vi "GetDefaultAcquisitionFileNames-subvi.vi"(0 "RAID root path":path=path "c:/scratch", 2 "Error In":errorcluster) -> (3 "last directory path":path, 4 "next directory path":path, 5 "all directory names":string[](array[string]), 6 "Error Out":errorcluster)   [LabVIEW 2014]
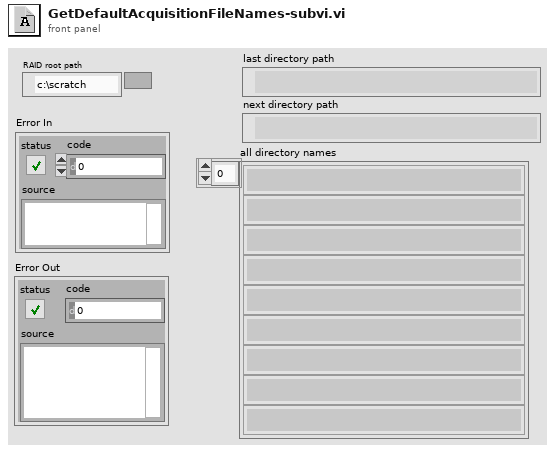
[diagram p1: front panel]
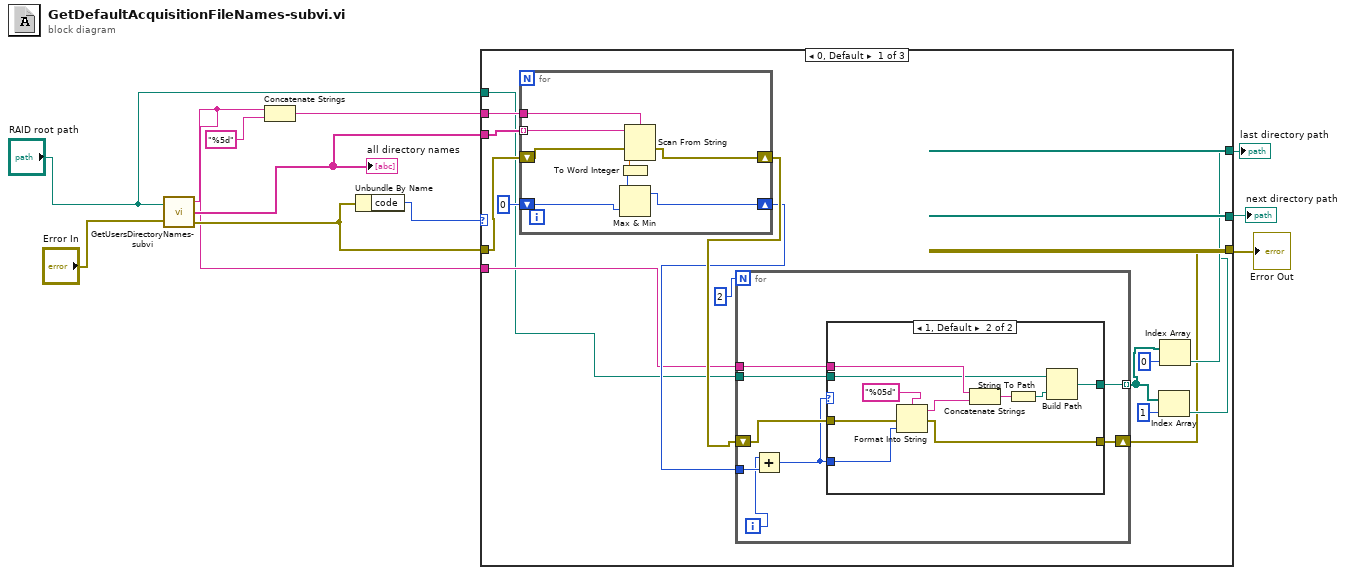
[diagram p0: block diagram]
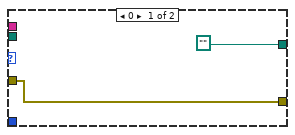
[diagram p2: hidden frame]
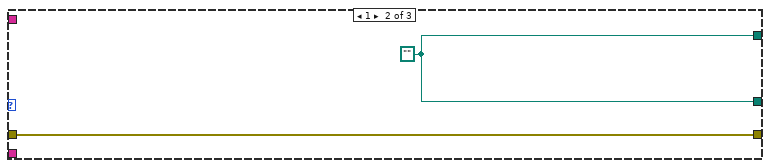
[diagram p3: hidden frame]
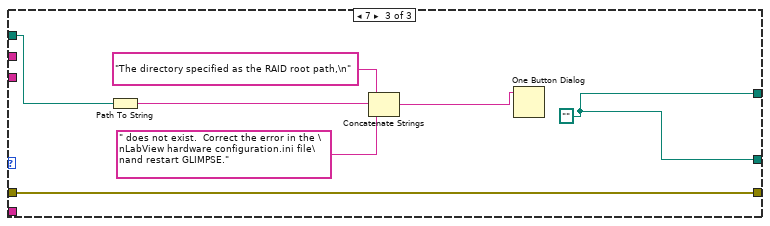
[diagram p4: hidden frame]
diagram:
  n1 = call "GetUsersDirectoryNames-subvi.vi"("RAID root path"="RAID root path", "Error In"="Error In") -> ("Username"=w5:string, "directory names"=w8:string[], "Error Out"=w6:errorcluster)
  "all directory names" <- w8
  n2 = Concatenate Strings(w5, "%5d" ("string")) -> (w9:string)
  n3 = Unbundle By Name(w6) -> ("code"=w7:i32)
  n4 = case shown="0, Default" w7 {
    tunnel: w9 -> [w25 _ _]
    tunnel: w8 -> [w24 _ _]
    tunnel: w6 -> [w23 w55 w58]
    tunnel: w5 -> [w19 _ _]
    tunnel: "RAID root path" -> [w18 _ w57]
    tunnel: [w14 w56 w59] -> w2
    tunnel: [w13 w56 w59] -> w1
    tunnel: [w12 w55 w58] -> w3
    frame 0, Default {
      n5 = for {
        shift-right: [w51] -> w21
        shift-left: 0 -> [w52]
        tunnel: w25 -> [w50]
        tunnel: w24 -> [w49] mode=indexing
        shift-right: [w47] -> w22
        shift-left: w23 -> [w48]
        n6 = Scan From String(format string=w50, input string=w49, error in=w48) -> (error out=w47:errorcluster, output 1=w53:dbl)  [unwired: 1 in, 3 out]
        n7 = To Word Integer(number=w53) -> (16bit integer=w54:i16)
        n8 = Max & Min(x=w54, y=w52) -> (max(x,y)=w51:i32)  [unwired: 1 out]
      }
      n9 = for {
        N: 2 -> [_]
        shift-right: [w27] -> w12
        shift-left: w22 -> [w32]
        tunnel: w21 -> [w34]
        tunnel: w19 -> [w30]
        tunnel: w18 -> [w29]
        tunnel: [w28] -> w15 mode=indexing
        i -> [w33]
        n10 = Add(x=w33, y=w34) -> (x+y=w31:i32)
        n11 = case shown="1, Default" w31 {
          tunnel: w32 -> [w36 w45]
          tunnel: w31 -> [_ w44]
          tunnel: w30 -> [_ w42]
          tunnel: w29 -> [_ w39]
          tunnel: [path "" w38] -> w28
          tunnel: [w36 w37] -> w27
          frame 0 {
          }
          frame 1, Default {
            n12 = Format Into String(format string="%05d", error in=w45, w44) -> (resulting string=w43:string, error out=w37:errorcluster)  [unwired: 1 in]
            n13 = Concatenate Strings(w42, w43) -> (w41:string)
            n14 = String To Path(string=w41) -> (path=w40:path)
            n15 = Build Path(base path=w39, name or relative path=w40) -> (appended path=w38:path)
          }
        }
      }
      n16 = Index Array(array=w15, index=1) -> (element=w13:path)
      n17 = Index Array(array=w15, index=0) -> (element=w14:path)
    }
    frame 1 {
      w56 = path ""
    }
    frame 7 {
      w59 = path ""
      n18 = Path To String(path=w57) -> (string=w63:string)
      n19 = Concatenate Strings("The directory specified as the RAID root path,\n", w63, " does not exist.  Correct the error in the \nLabView hardware configuration.ini file\nand restart GLIMPSE.") -> (w60:string)
      n20 = One Button Dialog(message=w60) -> ()  [unwired: 2 out]
    }
  }
  "Error Out" <- w3
  "next directory path" <- w1
  "last directory path" <- w2
